vi "Telnet Read.vi"(4 "line separator":string, 5 "read mode (normal)":enum16{"normal", "line", "buffered"}(ring), 6 "error in (no error)":errorcluster, 7 "timeout ms (25000)":i32=25000, 8 "bytes to read":i32=60, 9 "telnet connection":T1) -> (0 "error out":errorcluster, 2 "data out":string, 3 "telnet connection out":T1)   [LabVIEW 2015, in "NI_InternetTK_Core_VIs.lvlib"]
doc: "Reads data from a Telnet connection and returns the data after filtering out Telnet control characters."
uses:
  NI_InternetTK_Core_VIs.lvlib
  Telnet Session.ctl
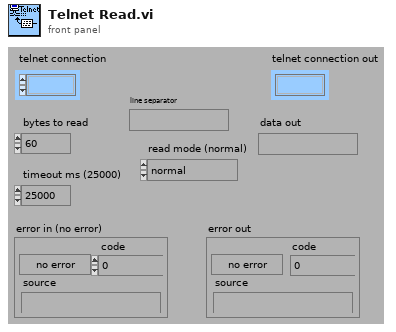
[diagram p1: front panel]
types:
  T1 = typedef "Telnet Session.ctl" = refnum<k1>
  T2 = enum16{"reset", "register", "get data", "set data", "unregister", "test", "get objects"}
  T3 = typedef "Telnet Connection Data.ctl" = cluster{"id":refnum<k5>, "read sem":T4, "write sem":T4, "read buffer":string, "read unfiltered buffer":string}
  T4 = typedef "__Semaphore RefNum" = refnum<k1>
  T5 = cluster{"bytes to read":i32, "timeout ms (25000)":i32, "read mode (normal)":enum16{"normal", "line", "buffered"}, "line separator":string}
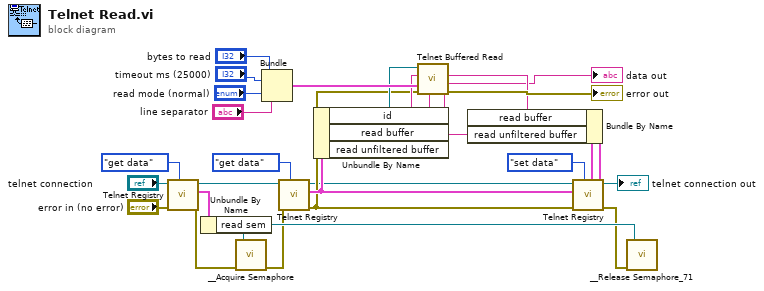
[diagram p0: block diagram]
diagram:
  n1 = call "Telnet Registry.vi"("function (get data)"=T2."get data", "error in (no error)"="error in (no error)", "object"="telnet connection") -> ("error out"=w19:errorcluster, "object data"=w15:T3, "object out"=w16:T1)  [unwired: 1 in, 5 out]
  n2 = Unbundle By Name(w15) -> ("read sem"=w20:T4)
  n3 = call "__Acquire Semaphore.vi"("error in (no error)"=w19, "semaphore"=w20) -> ("error out"=w9:errorcluster)  [unwired: 1 in, 4 out]
  n4 = Bundle("bytes to read"="bytes to read", "timeout ms (25000)"="timeout ms (25000)", "read mode (normal)"="read mode (normal)", "line separator"="line separator") -> (w26:T5)  [unwired: 1 out]
  n5 = call "Telnet Registry.vi"("function (get data)"=T2."get data", "error in (no error)"=w9, "object"=w16) -> ("error out"=w13:errorcluster, "object data"=w14:T3, "object out"=w11:T1)  [unwired: 1 in, 5 out]
  n6 = Unbundle By Name(w14) -> ("id"=w24:refnum<k5>, "read buffer"=w23:string, "read unfiltered buffer"=w4:string)
  n7 = call "Telnet Buffered Read.vi"("unfiltered buffer in"=w4, "error in (no error)"=w13, "read info"=w26, "buffer in"=w23, "connection ID"=w24) -> ("error out"=→"error out":errorcluster, "data"=→"data out":string, "buffer out"=w6:string, "unfiltered buffer out"=w3:string)  [unwired: 3 out]
  n8 = Bundle By Name(cluster=w14, "read buffer"=w6, "read unfiltered buffer"=w3) -> (w12:T3)
  n9 = call "Telnet Registry.vi"("function (get data)"=T2."set data", "error in (no error)"=w13, "object data in"=w12, "object"=w11) -> ("error out"=w8:errorcluster, "object out"=→"telnet connection out":T1)  [unwired: 6 out]
  n10 = call "__Release Semaphore_71.vi"("error in (no error)"=w8, "semaphore"=w20) -> ()  [unwired: 6 out]
